vi "GetCOMPort.vi"(9 "错误输入（无错误）":errorcluster, 10 "VISA引用句柄输入":refnum<visa-resource-name>) -> (1 "错误输出":errorcluster, 2 "Result":bool)   [LabVIEW 2013]
uses:
  <vilib>/Instr/_visa.llb/VISA Find Search Mode.ctl
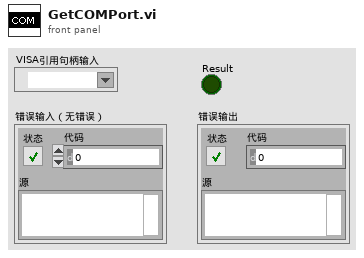
[diagram p1: front panel]
types:
  T1 = typedef "VISA Find Search Mode.ctl" = u32
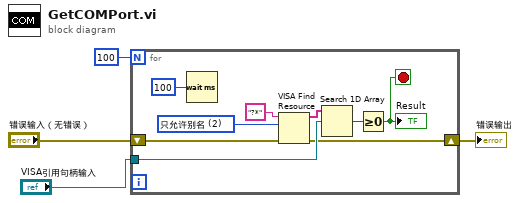
[diagram p0: block diagram]
diagram:
  n1 = for {
    N: 100 -> [_]
    tunnel: "VISA引用句柄输入" -> [w13]
    shift-right: [w5] -> w4
    shift-left: "错误输入（无错误）" -> [w6]
    stop <- w11 stop-if-true
    w10 = T1 2 items=["仅允许规范名称"=0, "只允许别名"=2, "包含匹配别名"=3, "包含所有别名"=4] ("Search Mode")
    n2 = Wait (ms)(milliseconds to wait=u32 100 ("等待时间（毫秒）")) -> ()  [unwired: 1 out]
    n3 = VISA Find Resource(8:w6, 10:w10, 11:"?*" ("表达式(\"?*\")")) -> (0:w5:errorcluster, 3:w8:string[])  [unwired: 1 out]
    n4 = Search 1D Array(1D array=w8, element=w13) -> (index of element=w12:i32)  [unwired: 1 in]
    n5 = Greater Or Equal To 0?(x=w12) -> (x >= 0?=w11:bool)
    "Result" <- w11
  }
  "错误输出" <- w4
